vi "cluster2array.vi"(11 "JSON":string) -> (1 "values":string[](array[string]), 2 "labels":string[](array[string]))   [LabVIEW 2014]
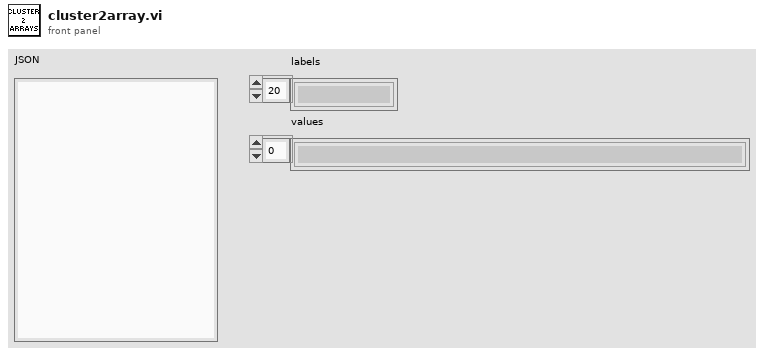
[diagram p1: front panel]
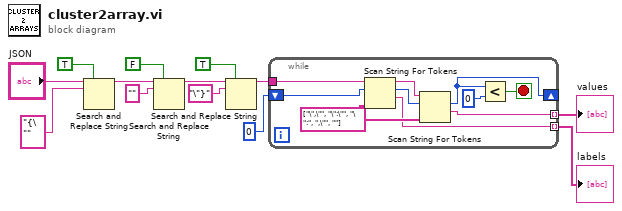
[diagram p0: block diagram]
diagram:
  n1 = Search and Replace String(replace all?=TRUE ("replace all? (F)"), input string="JSON", search string="{\"") -> (result string=w8:string)  [unwired: 5 in, 3 out]
  n2 = Search and Replace String(replace all?=FALSE ("replace all? (F)"), input string=w8, search string="") -> (result string=w5:string)  [unwired: 5 in, 3 out]
  n3 = Search and Replace String(replace all?=TRUE ("replace all? (F)"), input string=w5, search string="\"}") -> (result string=w1:string)  [unwired: 5 in, 3 out]
  n4 = while {
    shift-right: [w15] -> _
    shift-left: 0 ("offset past token") -> [w23]
    tunnel: [w19] -> w11 mode=indexing
    tunnel: [w18] -> w12 mode=indexing
    tunnel: w1 -> [w17]
    stop <- w16 stop-if-true
    w22 = string[] ["\",\"", "\":\"", "\":", ",\"", ""] ("delimiters (\\s,\\t,\\r,\\n)")
    n5 = Scan String For Tokens(6:w22, 8:w23, 9:w17) -> (1:w19:string, 2:w20:i32, 3:w21:string)  [unwired: 3 in, 1 out]
    n6 = Scan String For Tokens(6:w22, 8:w20, 9:w21) -> (1:w18:string, 2:w15:i32)  [unwired: 3 in, 2 out]
    n7 = Less?(x=w15, y=0) -> (x < y?=w16:bool)
  }
  "values" <- w12
  "labels" <- w11
